vi "Line Equation.vi"() -> ()   [LabVIEW 2019]
panel:
  in  "Enum":enum16{"Java", "Python", "C++", "Labview"}(ring)
  out "String 2":string
  in  "String":string
  out "Stop Button is pressed to stop the operation":bool
  in  "Stop the program":bool
  out "Slope (m) 2":dbl
  in  "Y-Intercept (b)":dbl
  in  "x":dbl
  in  "Slope (m)":dbl
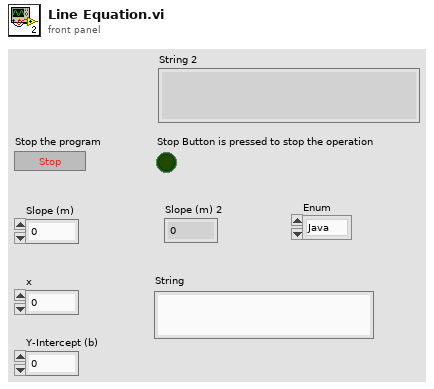
[diagram p1: front panel]
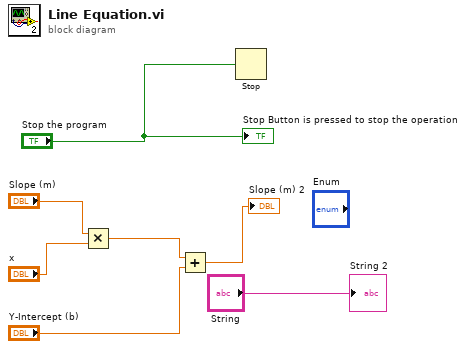
[diagram p0: block diagram]
diagram:
  n1 = Multiply(x="Slope (m)", y="x") -> (x*y=w5:dbl)
  n2 = Add(x=w5, y="Y-Intercept (b)") -> (x+y=→"Slope (m) 2":dbl)
  n3 = Stop(stop? (T)="Stop the program") -> ()
  "Stop Button is pressed to stop the operation" <- "Stop the program"
  "String 2" <- "String"
